vi "Initialize Analysis Workspace.vi"(8 "error in (no error)":errorcluster, 11 "reserved memory size (KB)":u32=2000) -> (0 "error out":errorcluster)   [LabVIEW 2017, in "NI_AALPro.lvlib"]
doc: "Initializes the analysis workspace on the RT target and sets the workspace size to <B>reserved memory size (KB)</B>. To prevent race conditions, priority inversions, and other undefined behavior, you must use the Initialize Analysis Workspace VI according to a strict set of guidelines."
uses:
  NI_AALPro.lvlib
  lvanlys.dll
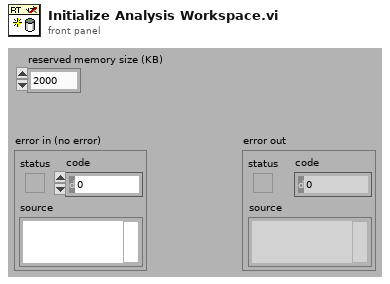
[diagram p1: front panel]
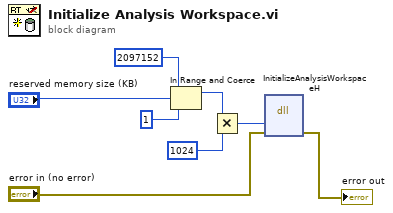
[diagram p0: block diagram]
diagram:
  n1 = In Range and Coerce(upper limit=u32 2097152, x="reserved memory size (KB)", lower limit=u32 1) -> (coerced(x)=w1:u32)  [unwired: 1 out]
  n2 = Multiply(x=w1, y=u32 1024) -> (x*y=w5:u32)
  n3 = dll-call lib="C:/Program Files/National Instruments/LabVIEW 2017/resource/lvanlys.*" fn="InitializeAnalysisWorkspaceH"("_sizeInKB"=w5, "_errorCluster"="error in (no error)") -> ("_errorCluster"=→"error out":errorcluster)  [unwired: 5 in, 2 out]
